vi "ObtainExpectedString.vi"(10 "Array":i8[](array[numeric])) -> (3 "detectedMessage":i8[](array[numeric]))   [LabVIEW 2022 SP3]
panel:
  out "CorrectComparisons":i32
  out "lastIteration":i8[](array[numeric])
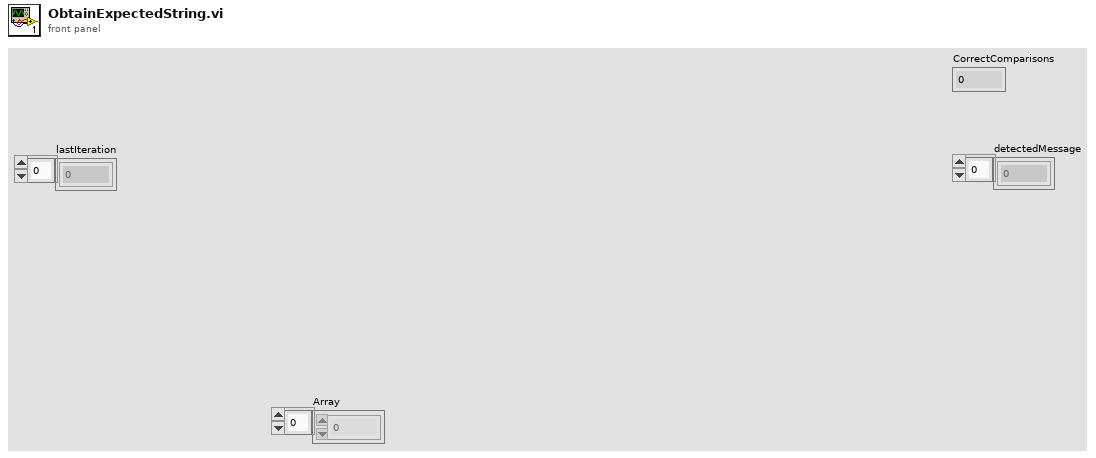
[diagram p1: front panel]
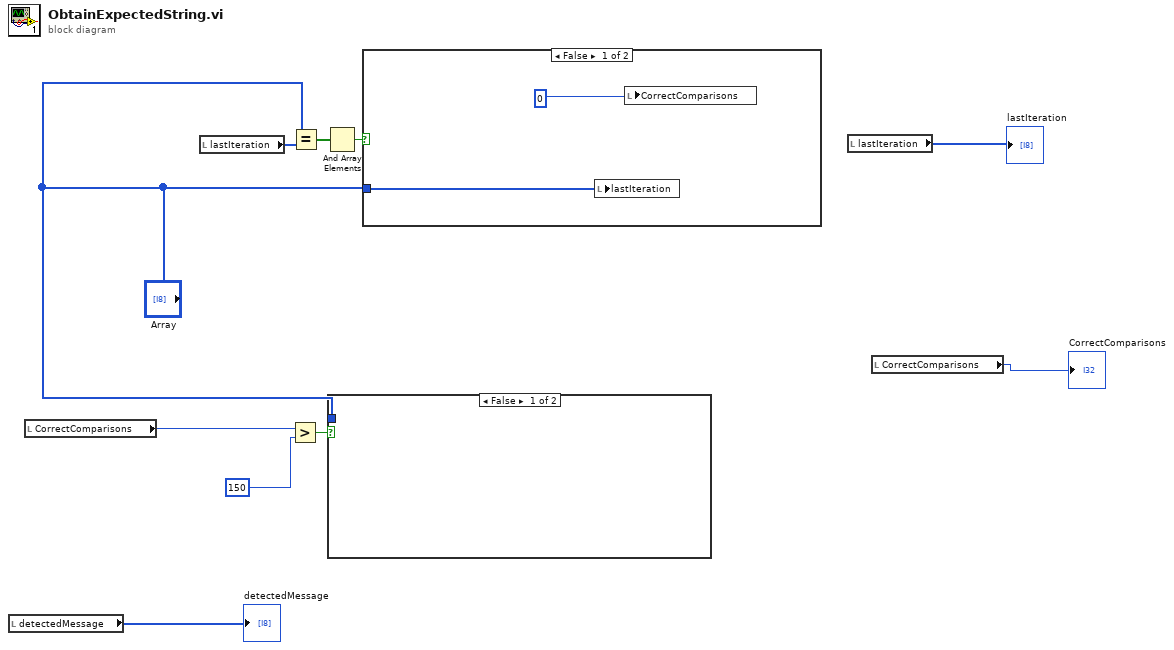
[diagram p0: block diagram]
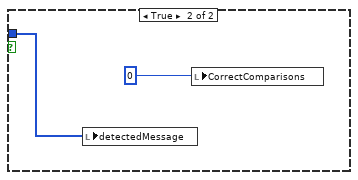
[diagram p2: hidden frame]
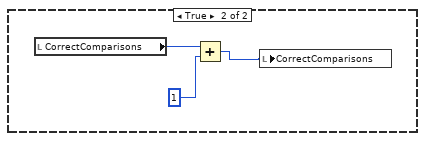
[diagram p3: hidden frame]
diagram:
  n1 = local read "detectedMessage"() -> (→"detectedMessage":i8[])
  n2 = local read "CorrectComparisons"() -> (w4:i32)
  n3 = local read "lastIteration"() -> (w10:i8[])
  n4 = Greater?(x=w4, y=150) -> (0:w6:bool)
  n5 = Equal?(x="Array", y=w10) -> (x = y?=w9:bool[])
  n6 = And Array Elements(Boolean array=w9) -> (logical AND=w8:bool)
  n7 = case shown="False" w6 {
    tunnel: "Array" -> [_ w12]
    frame False {
    }
    frame True {
      n8 = local write "detectedMessage"(w12) -> ()
      n9 = local write "CorrectComparisons"(0) -> ()
    }
  }
  n10 = case shown="False" w8 {
    tunnel: "Array" -> [w14 _]
    frame False {
      n11 = local write "lastIteration"(w14) -> ()
      n12 = local write "CorrectComparisons"(0) -> ()
    }
    frame True {
      n13 = local read "CorrectComparisons"() -> (w16:i32)
      n14 = Add(x=w16, y=1) -> (x+y=w15:i32)
      n15 = local write "CorrectComparisons"(w15) -> ()
    }
  }
  n16 = local read "lastIteration"() -> (→"lastIteration":i8[])
  n17 = local read "CorrectComparisons"() -> (→"CorrectComparisons":i32)
